vi "Initialize System.vi"(7 "physical channels":T5[](array[typedef]), 8 "error in (no error)":errorcluster, 9 "header":string, 10 "CFG-2":T1={"PMU ID"=1, "time base"=10000000, "nominal frequency"=enum."60 Hz", "reporting rate [fps]"=60, "station name"="", "data format"=15, "phasor channels"=[], "analog channels"=[], "digital channels"=[]} {"digital channels"."digital unit" format="%08x"; "analog channels"."analog unit" format="%08x"; "phasor channels"."phasor unit scaling" max=16777215 format="%06x"; "phasor channels"."phasor unit" items=["Voltage [V]"=0, "Current [A]"=16777216]; "data format" format="%016b"}, 11 "CFG-1":T1={"PMU ID"=1, "time base"=10000000, "nominal frequency"=enum."60 Hz", "reporting rate [fps]"=60, "station name"="", "data format"=15, "phasor channels"=[], "analog channels"=[], "digital channels"=[]} {"digital channels"."digital unit" format="%08x"; "analog channels"."analog unit" format="%08x"; "phasor channels"."phasor unit scaling" max=16777215 format="%06x"; "phasor channels"."phasor unit" items=["Voltage [V]"=0, "Current [A]"=16777216]; "data format" format="%016b"}) -> (0 "error out":errorcluster, 1 "system info out":refnum<class "PMU System Info.lvclass">, 3 "initial samples to read":u32=250)   [LabVIEW 2013, in "NI_EP_PMU.lvlib"]
doc: "LabVIEW no longer supports this VI. Use the Initialize System (Std 2011) VI instead.\n\nSets the basic configuration of a phasor measurement unit (PMU) system by specifying physical channels settings, configuration frame, and header frame according to IEEE Std C37.118:2005. This VI also returns the initial number of samples to read from DMA FIFOs."
uses:
  <vilib>/addons/Electrical Power/PMU/NI_EP_PMU.lvlib
  <vilib>/addons/Electrical Power/PMU/Common/Classes/PMU System Info/PMU System Info.lvclass
  <vilib>/addons/Electrical Power/PMU/Common/Controls/pmu_CFG Input.ctl
  <vilib>/addons/Electrical Power/PMU/Common/Controls/pmu_Phasor Channel.ctl
  <vilib>/addons/Electrical Power/PMU/Common/Controls/pmu_Analog Channel.ctl
  <vilib>/addons/Electrical Power/PMU/Common/Controls/pmu_Digital Channel.ctl
  <vilib>/addons/Electrical Power/PMU/Common/Controls/pmu_Physical Channel.ctl
  <vilib>/addons/Electrical Power/PMU/Common/Controls/pmu_Channel Phase.ctl
  <vilib>/addons/Electrical Power/PMU/Common/Controls/pmu_Frequency Detector Settings.ctl
  <vilib>/addons/Electrical Power/PMU/Common/Controls/pmu_ROCOF Detector Settings.ctl
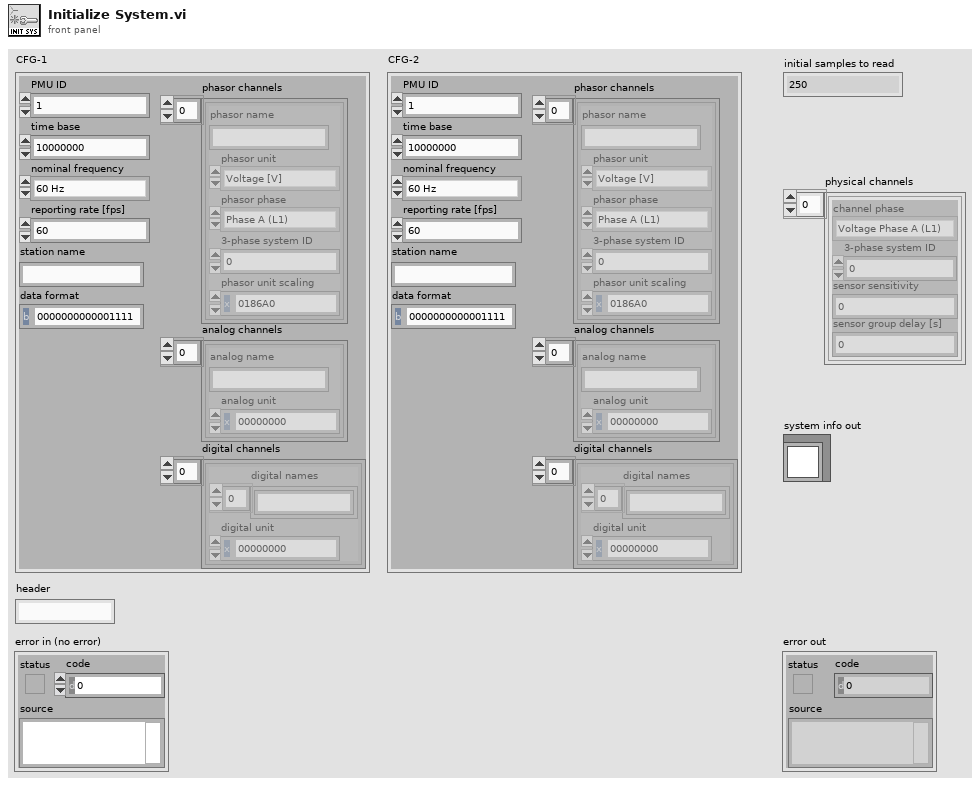
[diagram p1: front panel]
types:
  T1 = typedef "NI_EP_PMU.lvlib/pmu_CFG Input.ctl" = cluster{"PMU ID":u16, "time base":u32, "nominal frequency":enum16{"50 Hz", "60 Hz"}, "reporting rate [fps]":i16, "station name":string, "data format":u16, "phasor channels":T2[], "analog channels":T3[], "digital channels":T4[]}
  T2 = typedef "NI_EP_PMU.lvlib/pmu_Phasor Channel.ctl" = cluster{"phasor name":string, "phasor unit":u32, "phasor phase":enum16{"Phase A (L1)", "Phase B (L2)", "Phase C (L3)", "Phase N", "Positive sequence", "Negative sequence", "Zero sequence"}, "3-phase system ID":u8, "phasor unit scaling":u32}
  T3 = typedef "NI_EP_PMU.lvlib/pmu_Analog Channel.ctl" = cluster{"analog name":string, "analog unit":u32}
  T4 = typedef "NI_EP_PMU.lvlib/pmu_Digital Channel.ctl" = cluster{"digital names":string[], "digital unit":u32}
  T5 = typedef "NI_EP_PMU.lvlib/pmu_Physical Channel.ctl" = cluster{"channel phase":T6, "3-phase system ID":u8, "sensor sensitivity":dbl, "sensor group delay [s]":dbl}
  T6 = typedef "NI_EP_PMU.lvlib/pmu_Channel Phase.ctl" = enum16{"Voltage Phase A (L1)", "Voltage Phase B (L2)", "Voltage Phase C (L3)", "Voltage Phase N (Neutral)", "Current Phase A (L1)", "Current Phase B (L2)", "Current Phase C (L3)", "Current Phase N (Neutral)"}
  T7 = typedef "NI_EP_PMU.lvlib/pmu_ROCOF Detector Settings.ctl" = cluster{"ROCOF window width":i32}
  T8 = typedef "NI_EP_PMU.lvlib/pmu_Frequency Detector Settings.ctl" = cluster{"frequency window width":i32}
  T9 = typedef "NI_EP_PMU.lvlib/pmu_Phasor Channel Info.ctl" = cluster{"channel indexes":i32[], "phasor phase":enum16{"Phase A (L1)", "Phase B (L2)", "Phase C (L3)", "Phase N", "Positive sequence", "Negative sequence", "Zero sequence"}}
  T10 = typedef "NI_EP_PMU.lvlib/pmu_CFG Class.ctl" = cluster{"station name":string, "PMU ID":u16, "time base":u32, "nominal frequency":enum16{"50 Hz", "60 Hz"}, "reporting rate":i16, "phasor number":u16, "analog number":u16, "digital number":u16, "channel names":string[], "phasor units":u32[], "analog units":u32[], "digital units":u32[], "data format":u16, "number of PMUs":u16}
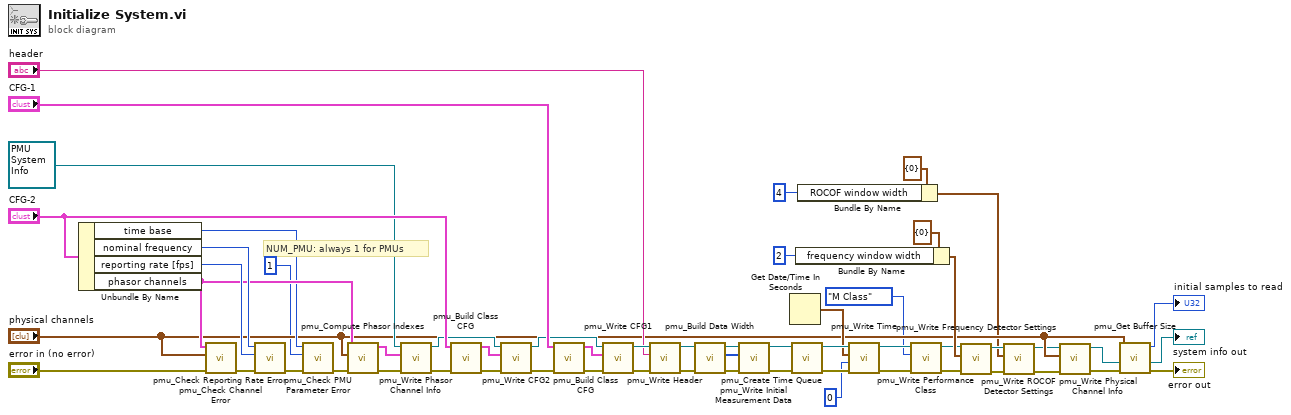
[diagram p0: block diagram]
diagram:
  # "NUM_PMU: always 1 for PMUs"
  n1 = Unbundle By Name("CFG-2") -> ("time base"=w34:u32, "nominal frequency"=w44:enum16{"50 Hz", "60 Hz"}, "reporting rate [fps]"=w43:i16, "phasor channels"=w42:T2[])
  n2 = call <vilib>:"pmu_Check Channel Error.vi"("error in (no error)"="error in (no error)", "physical channels"="physical channels", "phasor channels"=w42) -> ("error out"=w45:errorcluster)  [unwired: 8 in]
  n3 = call <vilib>:"pmu_Check Reporting Rate Error.vi"("error in (no error)"=w45, "reporting rate"=w43, "nominal frequency"=w44) -> ("error out"=w36:errorcluster)  [unwired: 8 in]
  n4 = call <vilib>:"pmu_Check PMU Parameter Error.vi"("error in (no error)"=w36, "number of PMUs"=u16 1, "time base"=w34) -> ("error out"=w35:errorcluster)  [unwired: 8 in]
  n5 = call <vilib>:"pmu_Compute Phasor Indexes.vi"("error in (no error)"=w35, "physical channels"="physical channels", "phasor channels"=w42) -> ("error out"=w41:errorcluster, "phasor channel info"=w39:T9[])  [unwired: 7 in]
  n6 = call <vilib>:"pmu_Write Phasor Channel Info.vi"("error in (no error)"=w41, "phasor channel info"=w39, "system info in"=refnum<class "PMU System Info.lvclass"> refnum ("PMU System Info.lvclass")) -> ("error out"=w40:errorcluster, "system info out"=w38:refnum<class "PMU System Info.lvclass">)  [unwired: 7 in]
  n7 = call <vilib>:"pmu_Build Class CFG.vi"("error in (no error)"=w40, "CFG input"="CFG-2") -> ("error out"=w49:errorcluster, "CFG class"=w50:T10)  [unwired: 8 in]
  n8 = call <vilib>:"pmu_Write CFG2.vi"("error in (no error)"=w49, "CFG-2"=w50, "system info in"=w38) -> ("error out"=w48:errorcluster, "system info out"=w47:refnum<class "PMU System Info.lvclass">)  [unwired: 7 in]
  n9 = call <vilib>:"pmu_Build Class CFG.vi"("error in (no error)"=w48, "CFG input"="CFG-1") -> ("error out"=w52:errorcluster, "CFG class"=w56:T10)  [unwired: 8 in]
  n10 = call <vilib>:"pmu_Write CFG1.vi"("error in (no error)"=w52, "CFG-1"=w56, "system info in"=w47) -> ("error out"=w28:errorcluster, "system info out"=w30:refnum<class "PMU System Info.lvclass">)  [unwired: 7 in]
  n11 = call <vilib>:"pmu_Write Header.vi"("error in (no error)"=w28, "header"="header", "system info in"=w30) -> ("error out"=w27:errorcluster, "system info out"=w29:refnum<class "PMU System Info.lvclass">)  [unwired: 7 in]
  n12 = call <vilib>:"pmu_Build Data Width.vi"("error in (no error)"=w27, "system info in"=w29) -> ("error out"=w31:errorcluster, "init meas data"=w32:u8[], "system info out"=w33:refnum<class "PMU System Info.lvclass">)  [unwired: 7 in]
  n13 = call <vilib>:"pmu_Write Initial Measurement Data.vi"("error in (no error)"=w31, "init meas data"=w32, "system info in"=w33) -> ("error out"=w24:errorcluster, "system info out"=w25:refnum<class "PMU System Info.lvclass">)  [unwired: 7 in]
  n14 = Get Date/Time In Seconds() -> (seconds since 1Jan1904=w21:timestamp)
  n15 = call <vilib>:"pmu_Create Time Queue.vi"("error in (no error)"=w24, "PMU System Info in"=w25) -> ("error out"=w22:errorcluster, "PMU System Info out"=w23:refnum<class "PMU System Info.lvclass">)  [unwired: 8 in]
  n16 = Bundle By Name(cluster=T8 {"frequency window width"=0} ("frequency detector settings"), "frequency window width"=2 ("window width")) -> (w17:T8)
  n17 = Bundle By Name(cluster=T7 {"ROCOF window width"=0} ("ROCOF detector settings"), "ROCOF window width"=4) -> (w2:T7)
  n18 = call <vilib>:"pmu_Write Time .vi"("error in (no error)"=w22, "time quality"=u8 0, "time stamp"=w21, "system info in"=w23) -> ("error out"=w9:errorcluster, "system info out"=w19:refnum<class "PMU System Info.lvclass">)  [unwired: 6 in]
  n19 = call <vilib>:"pmu_Write Performance Class.vi"("error in (no error)"=w9, "performance class"=enum8{"M Class", "P Class"}."M Class", "system info in"=w19) -> ("error out"=w8:errorcluster, "system info out"=w10:refnum<class "PMU System Info.lvclass">)  [unwired: 7 in]
  n20 = call <vilib>:"pmu_Write Frequency Detector Settings.vi"("error in (no error)"=w8, "frequency detector settings"=w17, "system info in"=w10) -> ("error out"=w5:errorcluster, "system info out"=w15:refnum<class "PMU System Info.lvclass">)  [unwired: 7 in]
  n21 = call <vilib>:"pmu_Write ROCOF Detector Settings.vi"("error in (no error)"=w5, "ROCOF detector settings"=w2, "system info in"=w15) -> ("error out"=w4:errorcluster, "system info out"=w6:refnum<class "PMU System Info.lvclass">)  [unwired: 7 in]
  n22 = call <vilib>:"pmu_Write Physical Channel Info.vi"("error in (no error)"=w4, "physical channels"="physical channels", "system info in"=w6) -> ("error out"=w12:errorcluster, "system info out"=w13:refnum<class "PMU System Info.lvclass">)  [unwired: 7 in]
  n23 = call <vilib>:"pmu_Get Buffer Size.vi"("error in (no error)"=w12, "PMU System Info in"=w13, "physical channels"="physical channels") -> ("error out"=→"error out":errorcluster, "PMU System Info out"=→"system info out":refnum<class "PMU System Info.lvclass">, "buffer size (samples)"=→"initial samples to read":u32)  [unwired: 6 in]
